vi "SwissSPAD Live_Settings Q.vi"() -> (5 "error out":errorcluster, 7 "Queue out":refnum<queue>)   [LabVIEW 2021]
uses:
  SwissSPAD Live_Settings Q Element.ctl
  SwissSPAD Live_Settings Q Action.ctl
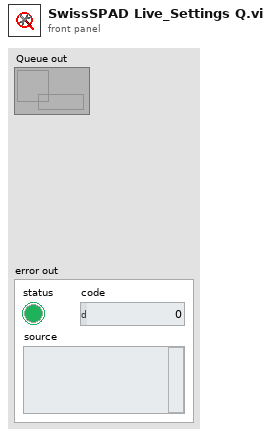
[diagram p1: front panel]
types:
  T1 = typedef "SwissSPAD Live_Settings Q Element.ctl" = cluster{"Action":T2, "Data":variant}
  T2 = typedef "SwissSPAD Live_Settings Q Action.ctl" = enum16{"Idle", "Initialization", "Refresh All Parameters", "Store Current Configuration", "Rename Current Configuration", "Delete Current Configuration", "Update Image ROI Information", "Load Hot Pixel Mask Image", "Quit"}
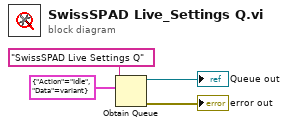
[diagram p0: block diagram]
diagram:
  n1 = Obtain Queue(name (unnamed)="SwissSPAD Live Settings Q", element data type=T1 {"Action"=enum."Idle", "Data"=variant} ("Settings Q Element")) -> (queue out=→"Queue out":refnum<queue>, error out=→"error out":errorcluster)  [unwired: 3 in, 1 out]
